vi "stop.vi"(8 "error in":errorcluster, 11 "Basic HTTP server in":refnum<class "Basic HTTPS server.lvclass">) -> (0 "error out":errorcluster)   [LabVIEW 2016, in "Basic HTTPS server.lvclass"]
uses:
  Basic HTTPS server.lvclass
  Basic HTTPS server.lvclass/Basic HTTPS server.ctl
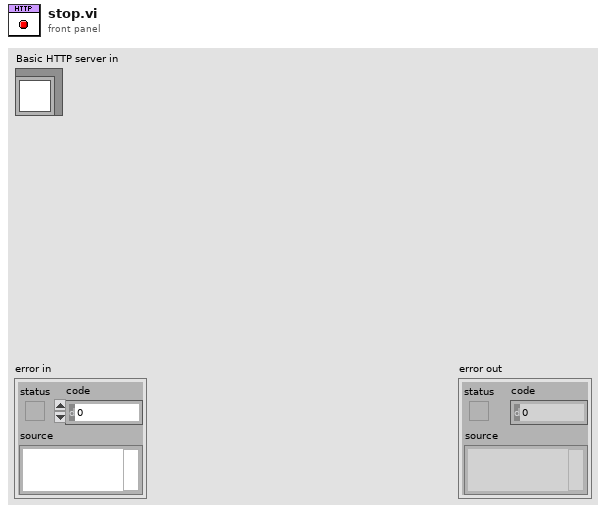
[diagram p1: front panel]
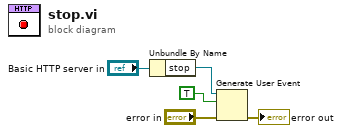
[diagram p0: block diagram]
diagram:
  n1 = Unbundle By Name("Basic HTTP server in") -> ("stop"=w2:refnum<user-event>)
  n2 = Generate User Event(user event=w2, event data cluster=TRUE ("event data"), error in="error in") -> (error out=→"error out":errorcluster)  [unwired: 1 in, 1 out]
